vi "data_to_string.vi"(10 "Camera":T2, 11 "Control Camera Properties 3":T1={"Packet Size"=1500, "Pixel Format"=17825797, "Gain in dB"=1.0, "Exposure Time in µs"=1500, "Stream Bytes per Second"=50000017} caption="Control Camera Properties" {"Stream Bytes per Second" min=1000000 max=124000000 step=100000 format="%.1p"; "Exposure Time in µs" min=21 max=153391689 format="%#.0f"; "Gain in dB" min=0.0 max=26.0 format="%#_2g"; "Pixel Format" items=["Mono 12 Packed"=17563654, "Mono 12"=17825797]}) -> (2 "Output string":string)   [LabVIEW 2014]
uses:
  type definitions/control camera properties.ctl
panel:
  # "Bytes"
  # "Trigger"
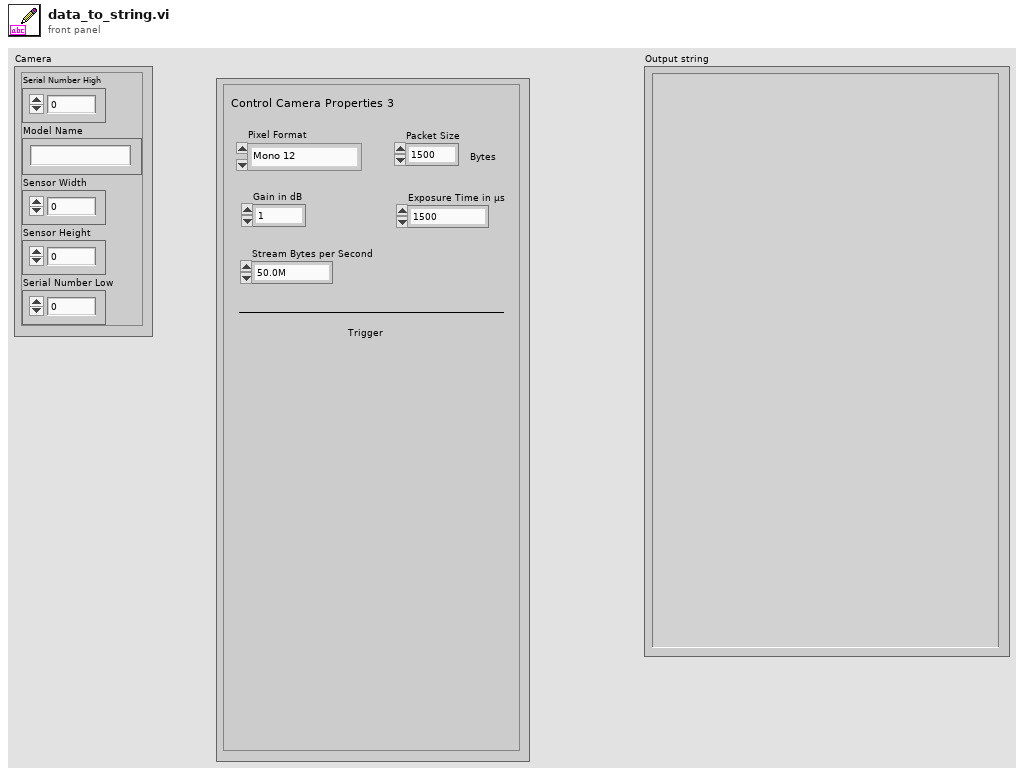
[diagram p1: front panel]
types:
  T1 = typedef "control camera properties.ctl" = cluster{"Packet Size":u32, "Pixel Format":u32, "Gain in dB":dbl, "Exposure Time in µs":u32, "Stream Bytes per Second":u32}
  T2 = cluster{"Serial Number High":u32, "Model Name":string, "Sensor Width":u32, "Sensor Height":u32, "Serial Number Low":u32}
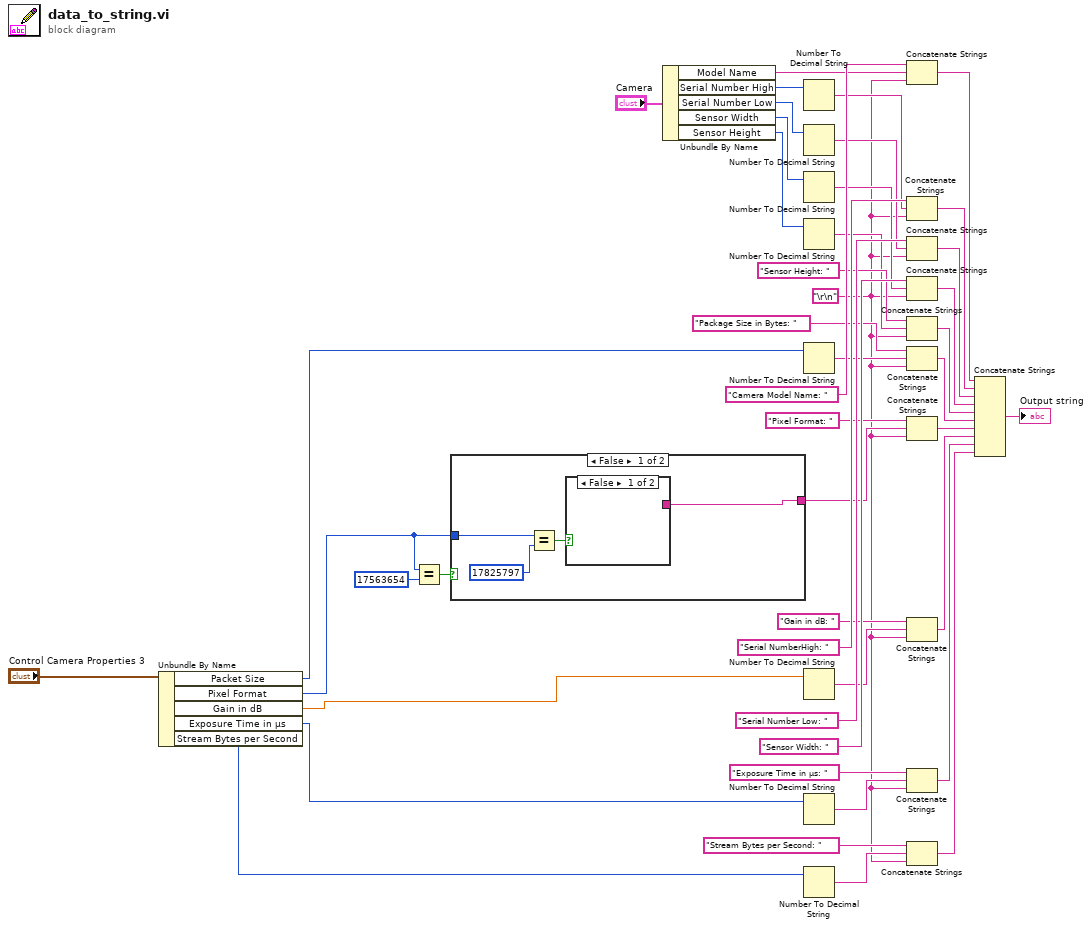
[diagram p0: block diagram]
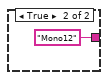
[diagram p2: hidden frame]
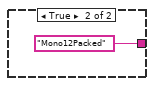
[diagram p3: hidden frame]
diagram:
  w7 = "\r\n"
  n1 = Unbundle By Name("Control Camera Properties 3") -> ("Packet Size"=w5:u32, "Pixel Format"=w4:u32, "Gain in dB"=w3:dbl, "Exposure Time in µs"=w2:u32, "Stream Bytes per Second"=w1:u32)
  n2 = Equal?(x=w4, y=u32 17563654) -> (x = y?=w39:bool)
  n3 = case shown="False" w39 {
    tunnel: w4 -> [w47 _]
    tunnel: [w46 "Mono12Packed"] -> w25
    frame False {
      n4 = Equal?(x=w47, y=u32 17825797) -> (x = y?=w49:bool)
      n5 = case shown="False" w49 {
        tunnel: [_ "Mono12"] -> w46
        frame False {
        }
        frame True {
        }
      }
    }
    frame True {
    }
  }
  n6 = Unbundle By Name("Camera") -> ("Model Name"=w35:string, "Serial Number High"=w44:u32, "Serial Number Low"=w43:u32, "Sensor Width"=w42:u32, "Sensor Height"=w41:u32)
  n7 = Number To Decimal String(number=w44) -> (decimal integer string=w36:string)  [unwired: 1 in]
  n8 = Number To Decimal String(number=w43) -> (decimal integer string=w33:string)  [unwired: 1 in]
  n9 = Number To Decimal String(number=w42) -> (decimal integer string=w31:string)  [unwired: 1 in]
  n10 = Number To Decimal String(number=w41) -> (decimal integer string=w29:string)  [unwired: 1 in]
  n11 = Number To Decimal String(number=w5) -> (decimal integer string=w28:string)  [unwired: 1 in]
  n12 = Number To Decimal String(number=w3) -> (decimal integer string=w23:string)  [unwired: 1 in]
  n13 = Number To Decimal String(number=w2) -> (decimal integer string=w21:string)  [unwired: 1 in]
  n14 = Number To Decimal String(number=w1) -> (decimal integer string=w19:string)  [unwired: 1 in]
  n15 = Concatenate Strings("Camera Model Name: ", w35, w7) -> (w17:string)
  n16 = Concatenate Strings("Serial NumberHigh: ", w36, w7) -> (w16:string)
  n17 = Concatenate Strings("Serial Number Low: ", w33, w7) -> (w15:string)
  n18 = Concatenate Strings("Sensor Width: ", w31, w7) -> (w14:string)
  n19 = Concatenate Strings("Sensor Height: ", w29, w7) -> (w13:string)
  n20 = Concatenate Strings("Package Size in Bytes: ", w28, w7) -> (w12:string)
  n21 = Concatenate Strings("Pixel Format: ", w25, w7) -> (w11:string)
  n22 = Concatenate Strings("Gain in dB: ", w23, w7) -> (w10:string)
  n23 = Concatenate Strings("Exposure Time in µs: ", w21, w7) -> (w9:string)
  n24 = Concatenate Strings("Stream Bytes per Second: ", w19, w7) -> (w8:string)
  n25 = Concatenate Strings(w17, w16, w15, w14, w13, w12, w11, w10, w9, w8) -> (→"Output string":string)
